vi "RichToFlatcif_manager_PluginInfoArray.vi"(5 "OutputClusterType":T1, 11 "InputCluster":T4) -> (3 "OutputCluster":T1)   [LabVIEW 2021, in "CIF_Manager_server.lvlib"]
uses:
  CIF_Manager_server.lvlib
  cif_manager_PluginInfoArray.ctl
  cif_manager_PluginInfo.ctl
  cif_manager_PluginVersion.ctl
  cif_manager_PluginInfoArray_Flat.ctl
  cif_manager_PluginInfo_Flat.ctl
  cif_manager_PluginVersion_Flat.ctl
  RichToFlatcif_manager_PluginVersion.vi
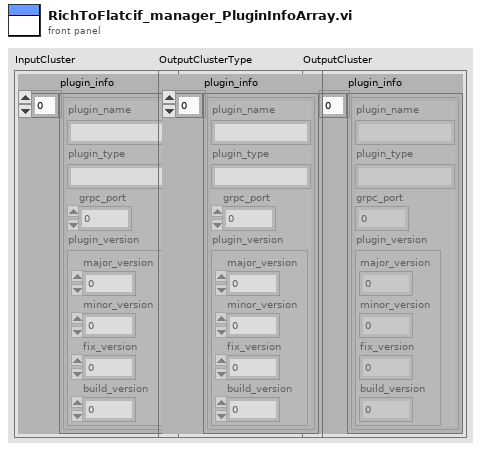
[diagram p1: front panel]
types:
  T1 = typedef "CIF_Manager_server.lvlib/cif_manager_PluginInfoArray_Flat.ctl" = cluster{"plugin_info":T2[]}
  T2 = typedef "CIF_Manager_server.lvlib/cif_manager_PluginInfo_Flat.ctl" = cluster{"plugin_name":string, "plugin_type":string, "grpc_port":i32, "plugin_version":T3}
  T3 = typedef "CIF_Manager_server.lvlib/cif_manager_PluginVersion_Flat.ctl" = cluster{"major_version":i32, "minor_version":i32, "fix_version":i32, "build_version":i32}
  T4 = typedef "CIF_Manager_server.lvlib/cif_manager_PluginInfoArray.ctl" = cluster{"plugin_info":T5[]}
  T5 = typedef "CIF_Manager_server.lvlib/cif_manager_PluginInfo.ctl" = cluster{"plugin_name":string, "plugin_type":string, "grpc_port":i32, "plugin_version":T6}
  T6 = typedef "CIF_Manager_server.lvlib/cif_manager_PluginVersion.ctl" = cluster{"major_version":i32, "minor_version":i32, "fix_version":i32, "build_version":i32}
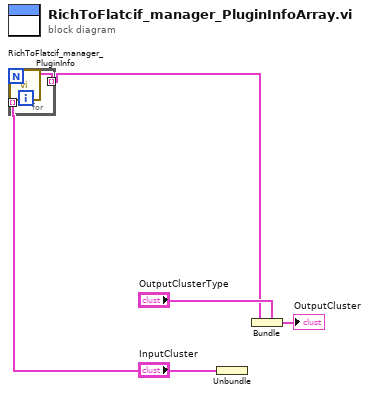
[diagram p0: block diagram]
diagram:
  n1 = Unbundle "Unbundle"("InputCluster") -> ("plugin_info"=w2:T5[])
  n2 = for {
    tunnel: w2 -> [w7] mode=indexing
    tunnel: [w6] -> w1 mode=indexing
    n3 = call "RichToFlatcif_manager_PluginInfo.vi"("InputCluster"=w7) -> ("OutputCluster"=w6:T2)  [unwired: 10 in]
  }
  n4 = Bundle "Bundle"(cluster="OutputClusterType", "plugin_info"=w1) -> (→"OutputCluster":T1)
